vi "ACal-Check Mic Level.vi"(9 "AI Waveforms in":dbl[][](array[numeric]), 11 "error in (no error)":errorcluster, 13 "Max Vmic":dbl) -> (10 "AI Waveforms out":dbl[][](array[numeric]), 15 "error out":errorcluster)   [LabVIEW 2020]
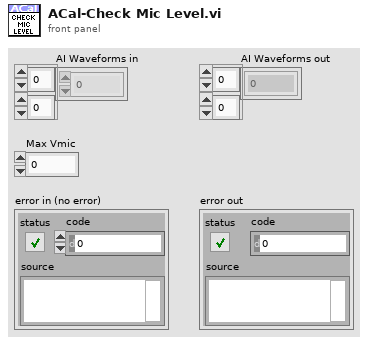
[diagram p1: front panel]
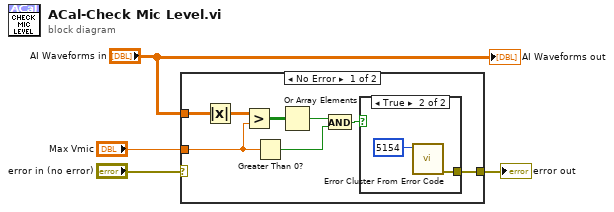
[diagram p0: block diagram]
diagram:
  n1 = case shown="No Error" "error in (no error)" {
    selector: "error in (no error)" -> [_ w15]
    tunnel: "AI Waveforms in" -> [w12 _]
    tunnel: "Max Vmic" -> [w6 _]
    tunnel: [w8 w15] -> w1
    frame No Error {
      n2 = Absolute Value(x=w12) -> (abs(x)=w11:dbl[][])
      n3 = Greater?(x=w11, y=w6) -> (0:w10:bool[][])
      n4 = Greater Than 0?(x=w6) -> (x > 0?=w5:bool)
      n5 = Or Array Elements(Boolean array=w10) -> (logical OR=w9:bool)
      n6 = And(x=w9, y=w5) -> (x .and. y?=w7:bool)
      n7 = case shown="True" w7 {
        tunnel: [_ w14] -> w8
        frame False {
        }
        frame True {
          n8 = call <vilib>:"Error Cluster From Error Code.vi"("error code (0)"=5154) -> ("error out"=w14:errorcluster)  [unwired: 8 in]
        }
      }
    }
    frame Error {
    }
  }
  "error out" <- w1
  "AI Waveforms out" <- "AI Waveforms in"
